vi "svc_Log View for Spectrum (MxN).vi"(0 "complex responses [EUy/EUx]":T9(array[cluster]) {"complex spectrum" format="%.2f"; "df" format="%.2f"; "f0" format="%.2f"}, 4 "spectra info in":T1[][](array[typedef]) {"x-axis units" items=["Time (s)"=0, "Frequency-CB (Hz)"=1, "Frequency-CPB (Hz)"=1248, "Frequency-Arbitrary (Hz)"=2357, "Quefrency (s)"=2, "Revolutions (rev)"=3, "Order"=4, "Speed (RPM)"=11, "Speed (rad/s)"=21, "Index"=65535]; "weighting filter" items=["Linear", "A-weighting", "B-weighting", "C-weighting", "ITU-R 468-4", "Dolby", "CCITT", "C-message", "Wb", "Wc", "Wd", "We", "Wf", "Wh", "Wj", "Wk", "Wm", "AES17 20 kHz lowpass", "AES17 40 kHz lowpass", "AES17 20 kHz highpass", "AES17 40 kHz highpass"]; "dB reference [EU]" format="%.2f"; "engineering units" items=["custom..."=0, "V"=1, "A"=21, "C"=30, "pC"=31, "s"=32, "-"=29, "Pa"=2, "N"=20, "g"=3, "m/s^2"=4, "m/s"=5, "m"=6, "mm/s"=12, "mm"=13, "micron/s"=14, "micron"=15, "in/s^2"=7, "in/s"=8, "in"=9, "mil/s"=10, "mil"=11, "rad/s^2"=16, "rad/s"=17, "rad"=18, "deg/s^2"=26, "deg/s"=27, "deg"=28, "RPM"=22, "cycle/s^2"=23, "Hz"=24, "cycle"=25, "strain"=19]; "spectral info"."window" items=["None "=0, "Hanning"=1, "Hamming"=2, "Blackman-Harris"=3, "Exact Blackman"=4, "Blackman"=5, "Flat Top"=6, "4 Term B-Harris "=7, "7 Term B-Harris"=8, "Low Sidelobe"=9, "Force - Exponential"=10, "Gaussian"=62]}, 5 "error in (no error)":errorcluster, 6 "view":enum16{"Mag-Phase", "Real-Imaginary"}(ring), 7 "view":T7={"dB On (T)"=TRUE, "unwrap phase (F)"=FALSE, "convert to degree (T)"=TRUE}) -> (12 "unit labels (mag or real)":string[][](array[string]), 13 "unit labels (phase or imag)":string[][](array[string]), 14 "magnitudes [dB EUy/EUx]":T8(array[cluster]) {"magnitude" format="%.2p"; "df" format="%.2p"; "f0" format="%.2p"}, 15 "phases [degree]":cluster{"f0":dbl, "df":dbl, "phase":dbl[]}[][](array[cluster]) {"phase" format="%.2f"; "df" format="%.2f"; "f0" format="%.2f"}, 18 "spectra info out":T1[][](array[typedef]) {"x-axis units" items=["Time (s)"=0, "Frequency-CB (Hz)"=1, "Frequency-CPB (Hz)"=1248, "Frequency-Arbitrary (Hz)"=2357, "Quefrency (s)"=2, "Revolutions (rev)"=3, "Order"=4, "Speed (RPM)"=11, "Speed (rad/s)"=21, "Index"=65535]; "weighting filter" items=["Linear", "A-weighting", "B-weighting", "C-weighting", "ITU-R 468-4", "Dolby", "CCITT", "C-message", "Wb", "Wc", "Wd", "We", "Wf", "Wh", "Wj", "Wk", "Wm", "AES17 20 kHz lowpass", "AES17 40 kHz lowpass", "AES17 20 kHz highpass", "AES17 40 kHz highpass"]; "dB reference [EU]" format="%.2f"; "engineering units" items=["custom..."=0, "V"=1, "A"=21, "C"=30, "pC"=31, "s"=32, "-"=29, "Pa"=2, "N"=20, "g"=3, "m/s^2"=4, "m/s"=5, "m"=6, "mm/s"=12, "mm"=13, "micron/s"=14, "micron"=15, "in/s^2"=7, "in/s"=8, "in"=9, "mil/s"=10, "mil"=11, "rad/s^2"=16, "rad/s"=17, "rad"=18, "deg/s^2"=26, "deg/s"=27, "deg"=28, "RPM"=22, "cycle/s^2"=23, "Hz"=24, "cycle"=25, "strain"=19]; "spectral info"."window" items=["None "=0, "Hanning"=1, "Hamming"=2, "Blackman-Harris"=3, "Exact Blackman"=4, "Blackman"=5, "Flat Top"=6, "4 Term B-Harris "=7, "7 Term B-Harris"=8, "Low Sidelobe"=9, "Force - Exponential"=10, "Gaussian"=62]}, 19 "error out":errorcluster)   [LabVIEW 2017]
uses:
  <vilib>/addons/_NISVFA/_Shared subVIs/Controls/svc_Spectrum Info.ctl
  <vilib>/addons/_NISVFA/_Shared subVIs/Controls/svc_X-Axis Units.ctl
  <vilib>/addons/_NISVFA/_Shared subVIs/Controls/svc_Spectrum Type.ctl
  <vilib>/addons/_NISVFA/_Shared subVIs/Controls/svc_Engineering Units Text Ring.ctl
  <vilib>/addons/_NISVFA/_Shared subVIs/Controls/svc_Weighting Filter Text Ring.ctl
  <vilib>/addons/_NISVFA/_Shared subVIs/Controls/svc_Complimentary Spectrum Units.ctl
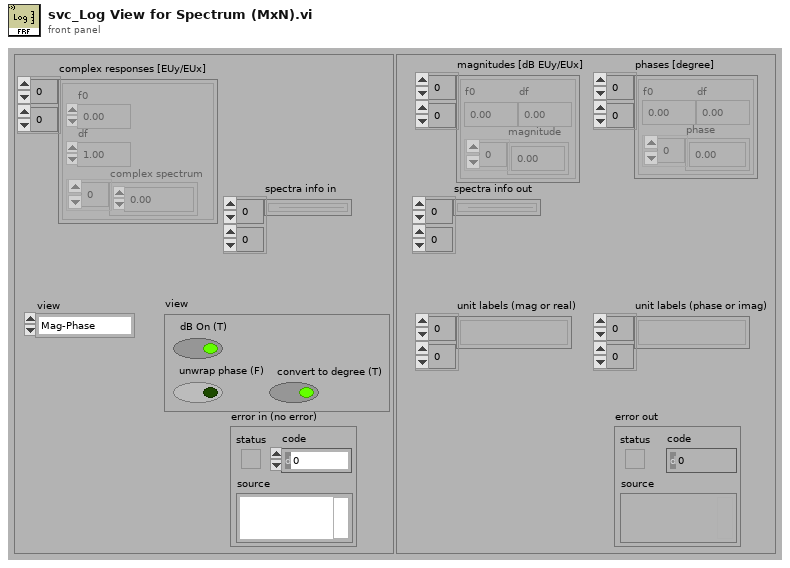
[diagram p1: front panel]
types:
  T1 = typedef "svc_Spectrum Info.ctl" = cluster{"channel name":string, "description":string, "x-axis units":T2, "spectral info":cluster{"spectrum type":T3, "linear/dB":enum16{"linear", "dB"}, "window":u16, "window size":i32, "FFT size":i32}, "engineering units":T4, "custom label":string, "dB reference [EU]":dbl, "peak units":enum16{"rms", "peak", "peak-peak"}, "weighting filter":T5, "spectral density?":bool, "unit label":string, "spectrum skewed?":bool, "complimentary spectrum units":T6}
  T2 = typedef "svc_X-Axis Units.ctl" = u16
  T3 = typedef "svc_Spectrum Type.ctl" = enum16{"FFT Spectrum [complex]", "Amplitude [Magnitude]", "Power [Magnitude^2]", "Cross Spectrum [complex]", "Frequency Response [Complex]"}
  T4 = typedef "svc_Engineering Units Text Ring.ctl" = u16
  T5 = typedef "svc_Weighting Filter Text Ring.ctl" = u16
  T6 = typedef "svc_Complimentary Spectrum Units.ctl" = enum16{"none", "radians", "degrees", "cycles", "imaginary"}
  T7 = cluster{"dB On (T)":bool, "unwrap phase (F)":bool, "convert to degree (T)":bool}
  T8 = cluster{"f0":dbl, "df":dbl, "magnitude":dbl[]}[][]
  T9 = cluster{"f0":dbl, "df":dbl, "complex spectrum":cdb[]}[][]
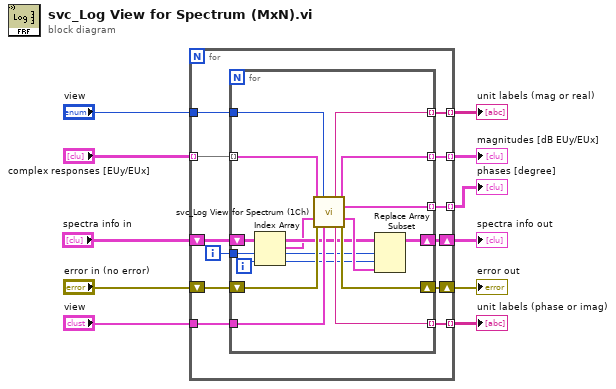
[diagram p0: block diagram]
diagram:
  n1 = for {
    tunnel: "complex responses [EUy/EUx]" -> [w23] mode=indexing
    tunnel: "view" -> [w22]
    tunnel: [w21] -> w9 mode=indexing
    tunnel: [w20] -> w8 mode=indexing
    tunnel: "view" -> [w19]
    tunnel: [w16] -> w4 mode=indexing
    tunnel: [w15] -> w3 mode=indexing
    shift-right: [w17] -> w5
    shift-left: "error in (no error)" -> [w18]
    shift-right: [w14] -> w2
    shift-left: "spectra info in" -> [w13]
    i -> [w12]
    n2 = for {
      tunnel: w23 -> [w30] mode=indexing
      tunnel: w22 -> [w38]
      tunnel: [w37] -> w21 mode=indexing
      tunnel: [w36] -> w20 mode=indexing
      tunnel: w19 -> [w35]
      tunnel: [w32] -> w16 mode=indexing
      tunnel: [w31] -> w15 mode=indexing
      shift-right: [w33] -> w17
      shift-left: w18 -> [w34]
      shift-right: [w26] -> w14
      shift-left: w13 -> [w25]
      tunnel: w12 -> [w28]
      i -> [w27]
      n3 = Index Array(array=w25, index (row)=w28, index (col)=w27) -> (element=w24:T1)
      n4 = call <vilib>:"svc_Log View for Spectrum (1Ch).vi"("complex spectrum"=w30, "View"=w38, "spectrum info in"=w24, "error in (no error)"=w34, "view"=w35) -> ("unit label [mag or real]"=w37:string, "magnitude or real"=w36:cluster{"f0":dbl, "df":dbl, dbl[]}, "phase or imag"=w32:cluster{"f0":dbl, "df":dbl, dbl[]}, "spectrum info out"=w29:T1, "unit label [phase or imag]"=w31:string, "error out"=w33:errorcluster)  [unwired: 5 in]
      n5 = Replace Array Subset(array=w25, new element=w29, index (row)=w28, index (col)=w27) -> (w26:T1[][])
    }
  }
  "unit labels (mag or real)" <- w9
  "magnitudes [dB EUy/EUx]" <- w8
  "error out" <- w5
  "phases [degree]" <- w4
  "unit labels (phase or imag)" <- w3
  "spectra info out" <- w2
